vi "Digital_Bridge_3_kart.vi"() -> ()   [LabVIEW 2014] (continued)
                                frame 9 {
                                n4367 = Index Array(array=w3016, index (row)=w3015, index (col)=w3014) -> (element=w3013:dbl)
                                n4368 = Replace Array Subset(array=w3016, new element=w3013, index (row)=w3015, index (col)=w3014) -> (w3017:dbl[][])
                                }
                                }
                                n4369 = local write "Denge Kosulu y1_y2"(w2957) -> ()
                                }
                              }
                              frame 4, Default {
                                n4370 = for {
                                N: 10 -> [_]
                                tunnel: w3018 -> [w3020]
                                i -> [w3023]
                                n4371 = local read "Denge Kosulu y1_y2"() -> (w3022:dbl[][])
                                n4372 = case shown="0, Default" w3023 {
                                tunnel: w3023 -> [w3025 w3030 w3038 w3043 w3048 w3053 w3057 w3064 w3070 w3075]
                                tunnel: w3022 -> [w3026 w3032 w3037 w3042 w3047 w3052 w3055 w3062 w3071 w3076]
                                tunnel: [w3027 w3033 w3035 w3041 w3046 w3051 w3054 w3061 w3072 w3077] -> w3021
                                tunnel: w3020 -> [w3028 w3031 w3036 w3040 w3045 w3050 w3056 w3063 w3069 w3074]
                                frame 0, Default {
                                n4373 = Index Array(array=w3026, index (row)=w3025, index (col)=w3028) -> (element=w3024:dbl)
                                n4374 = Replace Array Subset(array=w3026, new element=w3024, index (row)=w3025, index (col)=w3028) -> (w3027:dbl[][])
                                }
                                frame 1 {
                                n4375 = Index Array(array=w3032, index (row)=w3030, index (col)=w3031) -> (element=w3029:dbl)
                                n4376 = Replace Array Subset(array=w3032, new element=w3029, index (row)=w3030, index (col)=w3031) -> (w3033:dbl[][])
                                }
                                frame 2 {
                                n4377 = Index Array(array=w3037, index (row)=w3038, index (col)=w3036) -> (element=w3034:dbl)
                                n4378 = Replace Array Subset(array=w3037, new element=w3034, index (row)=w3038, index (col)=w3036) -> (w3035:dbl[][])
                                }
                                frame 3 {
                                n4379 = Index Array(array=w3042, index (row)=w3043, index (col)=w3040) -> (element=w3039:dbl)
                                n4380 = Replace Array Subset(array=w3042, new element=w3039, index (row)=w3043, index (col)=w3040) -> (w3041:dbl[][])
                                }
                                frame 4 {
                                n4381 = Index Array(array=w3047, index (row)=w3048, index (col)=w3045) -> (element=w3044:dbl)
                                n4382 = Replace Array Subset(array=w3047, new element=w3044, index (row)=w3048, index (col)=w3045) -> (w3046:dbl[][])
                                }
                                frame 5 {
                                n4383 = Index Array(array=w3052, index (row)=w3053, index (col)=w3050) -> (element=w3049:dbl)
                                n4384 = Replace Array Subset(array=w3052, new element=w3049, index (row)=w3053, index (col)=w3050) -> (w3051:dbl[][])
                                }
                                frame 6 {
                                n4385 = Index Array(array=w3055, index (row)=w3057, index (col)=w3056) -> (element=w3060:dbl)
                                n4386 = Multiply(x=w3060, y=2.0) -> (x*y=w3058:dbl)
                                n4387 = Replace Array Subset(array=w3055, new element=w3058, index (row)=w3057, index (col)=w3056) -> (w3054:dbl[][])
                                }
                                frame 7 {
                                n4388 = Index Array(array=w3062, index (row)=w3064, index (col)=w3063) -> (element=w3067:dbl)
                                n4389 = Multiply(x=w3067, y=2.0) -> (x*y=w3065:dbl)
                                n4390 = Replace Array Subset(array=w3062, new element=w3065, index (row)=w3064, index (col)=w3063) -> (w3061:dbl[][])
                                }
                                frame 8 {
                                n4391 = Index Array(array=w3071, index (row)=w3070, index (col)=w3069) -> (element=w3068:dbl)
                                n4392 = Replace Array Subset(array=w3071, new element=w3068, index (row)=w3070, index (col)=w3069) -> (w3072:dbl[][])
                                }
                                frame 9 {
                                n4393 = Index Array(array=w3076, index (row)=w3075, index (col)=w3074) -> (element=w3073:dbl)
                                n4394 = Replace Array Subset(array=w3076, new element=w3073, index (row)=w3075, index (col)=w3074) -> (w3077:dbl[][])
                                }
                                }
                                n4395 = local write "Denge Kosulu y1_y2"(w3021) -> ()
                                }
                              }
                              frame 5 {
                                n4396 = for {
                                N: 10 -> [_]
                                tunnel: w3078 -> [w3080]
                                i -> [w3083]
                                n4397 = local read "Denge Kosulu y1_y2"() -> (w3082:dbl[][])
                                n4398 = case shown="0, Default" w3083 {
                                tunnel: w3083 -> [w3084 w3091 w3102 w3107 w3112 w3117 w3122 w3127 w3132 w3136]
                                tunnel: w3082 -> [w3085 w3093 w3101 w3106 w3111 w3116 w3120 w3125 w3133 w3137]
                                tunnel: [w3086 w3094 w3099 w3105 w3110 w3115 w3119 w3124 w3134 w3138] -> w3081
                                tunnel: w3080 -> [w3087 w3092 w3100 w3104 w3109 w3114 w3121 w3126 w3131 w3135]
                                frame 0, Default {
                                n4399 = Index Array(array=w3085, index (row)=w3084, index (col)=w3087) -> (element=w3090:dbl)
                                n4400 = Multiply(x=w3090, y=2.0) -> (x*y=w3088:dbl)
                                n4401 = Replace Array Subset(array=w3085, new element=w3088, index (row)=w3084, index (col)=w3087) -> (w3086:dbl[][])
                                }
                                frame 1 {
                                n4402 = Index Array(array=w3093, index (row)=w3091, index (col)=w3092) -> (element=w3097:dbl)
                                n4403 = Multiply(x=w3097, y=2.0) -> (x*y=w3095:dbl)
                                n4404 = Replace Array Subset(array=w3093, new element=w3095, index (row)=w3091, index (col)=w3092) -> (w3094:dbl[][])
                                }
                                frame 2 {
                                n4405 = Index Array(array=w3101, index (row)=w3102, index (col)=w3100) -> (element=w3098:dbl)
                                n4406 = Replace Array Subset(array=w3101, new element=w3098, index (row)=w3102, index (col)=w3100) -> (w3099:dbl[][])
                                }
                                frame 3 {
                                n4407 = Index Array(array=w3106, index (row)=w3107, index (col)=w3104) -> (element=w3103:dbl)
                                n4408 = Replace Array Subset(array=w3106, new element=w3103, index (row)=w3107, index (col)=w3104) -> (w3105:dbl[][])
                                }
                                frame 4 {
                                n4409 = Index Array(array=w3111, index (row)=w3112, index (col)=w3109) -> (element=w3108:dbl)
                                n4410 = Replace Array Subset(array=w3111, new element=w3108, index (row)=w3112, index (col)=w3109) -> (w3110:dbl[][])
                                }
                                frame 5 {
                                n4411 = Index Array(array=w3116, index (row)=w3117, index (col)=w3114) -> (element=w3113:dbl)
                                n4412 = Replace Array Subset(array=w3116, new element=w3113, index (row)=w3117, index (col)=w3114) -> (w3115:dbl[][])
                                }
                                frame 6 {
                                n4413 = Index Array(array=w3120, index (row)=w3122, index (col)=w3121) -> (element=w3118:dbl)
                                n4414 = Replace Array Subset(array=w3120, new element=w3118, index (row)=w3122, index (col)=w3121) -> (w3119:dbl[][])
                                }
                                frame 7 {
                                n4415 = Index Array(array=w3125, index (row)=w3127, index (col)=w3126) -> (element=w3123:dbl)
                                n4416 = Replace Array Subset(array=w3125, new element=w3123, index (row)=w3127, index (col)=w3126) -> (w3124:dbl[][])
                                }
                                frame 8 {
                                n4417 = Index Array(array=w3133, index (row)=w3132, index (col)=w3131) -> (element=w3130:dbl)
                                n4418 = Multiply(x=w3130, y=2.0) -> (x*y=w3128:dbl)
                                n4419 = Replace Array Subset(array=w3133, new element=w3128, index (row)=w3132, index (col)=w3131) -> (w3134:dbl[][])
                                }
                                frame 9 {
                                n4420 = Index Array(array=w3137, index (row)=w3136, index (col)=w3135) -> (element=w3141:dbl)
                                n4421 = Multiply(x=w3141, y=2.0) -> (x*y=w3139:dbl)
                                n4422 = Replace Array Subset(array=w3137, new element=w3139, index (row)=w3136, index (col)=w3135) -> (w3138:dbl[][])
                                }
                                }
                                n4423 = local write "Denge Kosulu y1_y2"(w3081) -> ()
                                }
                              }
                            }
                          }
                        }
                        n4424 = Equal?(x=w2179, y=0.0) -> (x = y?=w2177:bool)
                        n4425 = case shown="True" w2177 {
                          tunnel: [w2182 w2184] -> w2176
                          frame False {
                            n4426 = local read "frekans index"() -> (w2183:dbl)
                            n4427 = Decrement(x=w2183) -> (x-1=w2182:dbl)
                          }
                          frame True {
                            n4428 = local read "Frekanslar"() -> (w2186:dbl[])
                            n4429 = Array Size(array=w2186) -> (size(s)=w2187:i32)
                            n4430 = Decrement(x=w2187) -> (x-1=w2185:i32)
                            n4431 = To Double Precision Float(number=w2185) -> (double precision float=w2184:dbl)
                          }
                        }
                      }
                      frame True {
                        n4432 = flat-sequence {
                          tunnel: w3142 -> [w3155]
                          tunnel: [w3155] -> w3147
                          tunnel: w3147 -> [w3476]
                          tunnel: [w3476] -> w3146
                          tunnel: w3146 -> [w3797]
                          frame #0 {
                            n4433 = for {
                              N: 5 -> [_]
                              tunnel: w3155 -> [w3158]
                              i -> [w3157]
                              n4434 = Increment(x=w3157) -> (x+1=w3156:i32)
                              n4435 = case shown="1" w3156 {
                                tunnel: w3158 -> [w3159 w3223 w3287 w3351 w3411]
                                frame 1 {
                                n4436 = for {
                                N: 10 -> [_]
                                tunnel: w3159 -> [w3161]
                                i -> [w3164]
                                n4437 = local read "Denge Kosulu x2_y2"() -> (w3163:dbl[][])
                                n4438 = case shown="5" w3164 {
                                tunnel: w3164 -> [w3165 w3172 w3183 w3188 w3193 w3198 w3203 w3208 w3213 w3217]
                                tunnel: w3163 -> [w3166 w3174 w3182 w3187 w3192 w3197 w3201 w3206 w3214 w3218]
                                tunnel: [w3167 w3175 w3180 w3186 w3191 w3196 w3200 w3205 w3215 w3219] -> w3162
                                tunnel: w3161 -> [w3168 w3173 w3181 w3185 w3190 w3195 w3202 w3207 w3212 w3216]
                                frame 0, Default {
                                n4439 = Index Array(array=w3166, index (row)=w3165, index (col)=w3168) -> (element=w3171:dbl)
                                n4440 = Multiply(x=w3171, y=2.0) -> (x*y=w3169:dbl)
                                n4441 = Replace Array Subset(array=w3166, new element=w3169, index (row)=w3165, index (col)=w3168) -> (w3167:dbl[][])
                                }
                                frame 1 {
                                n4442 = Index Array(array=w3174, index (row)=w3172, index (col)=w3173) -> (element=w3178:dbl)
                                n4443 = Multiply(x=w3178, y=2.0) -> (x*y=w3176:dbl)
                                n4444 = Replace Array Subset(array=w3174, new element=w3176, index (row)=w3172, index (col)=w3173) -> (w3175:dbl[][])
                                }
                                frame 2 {
                                n4445 = Index Array(array=w3182, index (row)=w3183, index (col)=w3181) -> (element=w3179:dbl)
                                n4446 = Replace Array Subset(array=w3182, new element=w3179, index (row)=w3183, index (col)=w3181) -> (w3180:dbl[][])
                                }
                                frame 3 {
                                n4447 = Index Array(array=w3187, index (row)=w3188, index (col)=w3185) -> (element=w3184:dbl)
                                n4448 = Replace Array Subset(array=w3187, new element=w3184, index (row)=w3188, index (col)=w3185) -> (w3186:dbl[][])
                                }
                                frame 4 {
                                n4449 = Index Array(array=w3192, index (row)=w3193, index (col)=w3190) -> (element=w3189:dbl)
                                n4450 = Replace Array Subset(array=w3192, new element=w3189, index (row)=w3193, index (col)=w3190) -> (w3191:dbl[][])
                                }
                                frame 5 {
                                n4451 = Index Array(array=w3197, index (row)=w3198, index (col)=w3195) -> (element=w3194:dbl)
                                n4452 = Replace Array Subset(array=w3197, new element=w3194, index (row)=w3198, index (col)=w3195) -> (w3196:dbl[][])
                                }
                                frame 6 {
                                n4453 = Index Array(array=w3201, index (row)=w3203, index (col)=w3202) -> (element=w3199:dbl)
                                n4454 = Replace Array Subset(array=w3201, new element=w3199, index (row)=w3203, index (col)=w3202) -> (w3200:dbl[][])
                                }
                                frame 7 {
                                n4455 = Index Array(array=w3206, index (row)=w3208, index (col)=w3207) -> (element=w3204:dbl)
                                n4456 = Replace Array Subset(array=w3206, new element=w3204, index (row)=w3208, index (col)=w3207) -> (w3205:dbl[][])
                                }
                                frame 8 {
                                n4457 = Index Array(array=w3214, index (row)=w3213, index (col)=w3212) -> (element=w3211:dbl)
                                n4458 = Multiply(x=w3211, y=2.0) -> (x*y=w3209:dbl)
                                n4459 = Replace Array Subset(array=w3214, new element=w3209, index (row)=w3213, index (col)=w3212) -> (w3215:dbl[][])
                                }
                                frame 9 {
                                n4460 = Index Array(array=w3218, index (row)=w3217, index (col)=w3216) -> (element=w3222:dbl)
                                n4461 = Multiply(x=w3222, y=2.0) -> (x*y=w3220:dbl)
                                n4462 = Replace Array Subset(array=w3218, new element=w3220, index (row)=w3217, index (col)=w3216) -> (w3219:dbl[][])
                                }
                                }
                                n4463 = local write "Denge Kosulu x2_y2"(w3162) -> ()
                                }
                                }
                                frame 2 {
                                n4464 = for {
                                N: 10 -> [_]
                                tunnel: w3223 -> [w3225]
                                i -> [w3228]
                                n4465 = local read "Denge Kosulu x2_y2"() -> (w3227:dbl[][])
                                n4466 = case shown="7" w3228 {
                                tunnel: w3228 -> [w3230 w3235 w3242 w3249 w3256 w3263 w3271 w3276 w3279 w3284]
                                tunnel: w3227 -> [w3231 w3237 w3241 w3248 w3255 w3262 w3269 w3274 w3280 w3285]
                                tunnel: [w3232 w3238 w3239 w3247 w3254 w3261 w3268 w3273 w3281 w3286] -> w3226
                                tunnel: w3225 -> [w3233 w3236 w3240 w3246 w3253 w3260 w3270 w3275 w3278 w3283]
                                frame 0, Default {
                                n4467 = Index Array(array=w3231, index (row)=w3230, index (col)=w3233) -> (element=w3229:dbl)
                                n4468 = Replace Array Subset(array=w3231, new element=w3229, index (row)=w3230, index (col)=w3233) -> (w3232:dbl[][])
                                }
                                frame 1 {
                                n4469 = Index Array(array=w3237, index (row)=w3235, index (col)=w3236) -> (element=w3234:dbl)
                                n4470 = Replace Array Subset(array=w3237, new element=w3234, index (row)=w3235, index (col)=w3236) -> (w3238:dbl[][])
                                }
                                frame 2 {
                                n4471 = Index Array(array=w3241, index (row)=w3242, index (col)=w3240) -> (element=w3245:dbl)
                                n4472 = Multiply(x=w3245, y=2.0) -> (x*y=w3243:dbl)
                                n4473 = Replace Array Subset(array=w3241, new element=w3243, index (row)=w3242, index (col)=w3240) -> (w3239:dbl[][])
                                }
                                frame 3 {
                                n4474 = Index Array(array=w3248, index (row)=w3249, index (col)=w3246) -> (element=w3252:dbl)
                                n4475 = Multiply(x=w3252, y=2.0) -> (x*y=w3250:dbl)
                                n4476 = Replace Array Subset(array=w3248, new element=w3250, index (row)=w3249, index (col)=w3246) -> (w3247:dbl[][])
                                }
                                frame 4 {
                                n4477 = Index Array(array=w3255, index (row)=w3256, index (col)=w3253) -> (element=w3259:dbl)
                                n4478 = Multiply(x=w3259, y=2.0) -> (x*y=w3257:dbl)
                                n4479 = Replace Array Subset(array=w3255, new element=w3257, index (row)=w3256, index (col)=w3253) -> (w3254:dbl[][])
                                }
                                frame 5 {
                                n4480 = Index Array(array=w3262, index (row)=w3263, index (col)=w3260) -> (element=w3266:dbl)
                                n4481 = Multiply(x=w3266, y=2.0) -> (x*y=w3264:dbl)
                                n4482 = Replace Array Subset(array=w3262, new element=w3264, index (row)=w3263, index (col)=w3260) -> (w3261:dbl[][])
                                }
                                frame 6 {
                                n4483 = Index Array(array=w3269, index (row)=w3271, index (col)=w3270) -> (element=w3267:dbl)
                                n4484 = Replace Array Subset(array=w3269, new element=w3267, index (row)=w3271, index (col)=w3270) -> (w3268:dbl[][])
                                }
                                frame 7 {
                                n4485 = Index Array(array=w3274, index (row)=w3276, index (col)=w3275) -> (element=w3272:dbl)
                                n4486 = Replace Array Subset(array=w3274, new element=w3272, index (row)=w3276, index (col)=w3275) -> (w3273:dbl[][])
                                }
                                frame 8 {
                                n4487 = Index Array(array=w3280, index (row)=w3279, index (col)=w3278) -> (element=w3277:dbl)
                                n4488 = Replace Array Subset(array=w3280, new element=w3277, index (row)=w3279, index (col)=w3278) -> (w3281:dbl[][])
                                }
                                frame 9 {
                                n4489 = Index Array(array=w3285, index (row)=w3284, index (col)=w3283) -> (element=w3282:dbl)
                                n4490 = Replace Array Subset(array=w3285, new element=w3282, index (row)=w3284, index (col)=w3283) -> (w3286:dbl[][])
                                }
                                }
                                n4491 = local write "Denge Kosulu x2_y2"(w3226) -> ()
                                }
                                }
                                frame 3 {
                                n4492 = for {
                                N: 10 -> [_]
                                tunnel: w3287 -> [w3289]
                                i -> [w3292]
                                n4493 = local read "Denge Kosulu x2_y2"() -> (w3291:dbl[][])
                                n4494 = case shown="6" w3292 {
                                tunnel: w3292 -> [w3294 w3299 w3306 w3313 w3320 w3327 w3335 w3340 w3343 w3348]
                                tunnel: w3291 -> [w3295 w3301 w3305 w3312 w3319 w3326 w3333 w3338 w3344 w3349]
                                tunnel: [w3296 w3302 w3303 w3311 w3318 w3325 w3332 w3337 w3345 w3350] -> w3290
                                tunnel: w3289 -> [w3297 w3300 w3304 w3310 w3317 w3324 w3334 w3339 w3342 w3347]
                                frame 0, Default {
                                n4495 = Index Array(array=w3295, index (row)=w3294, index (col)=w3297) -> (element=w3293:dbl)
                                n4496 = Replace Array Subset(array=w3295, new element=w3293, index (row)=w3294, index (col)=w3297) -> (w3296:dbl[][])
                                }
                                frame 1 {
                                n4497 = Index Array(array=w3301, index (row)=w3299, index (col)=w3300) -> (element=w3298:dbl)
                                n4498 = Replace Array Subset(array=w3301, new element=w3298, index (row)=w3299, index (col)=w3300) -> (w3302:dbl[][])
                                }
                                frame 2 {
                                n4499 = Index Array(array=w3305, index (row)=w3306, index (col)=w3304) -> (element=w3309:dbl)
                                n4500 = Multiply(x=w3309, y=2.0) -> (x*y=w3307:dbl)
                                n4501 = Replace Array Subset(array=w3305, new element=w3307, index (row)=w3306, index (col)=w3304) -> (w3303:dbl[][])
                                }
                                frame 3 {
                                n4502 = Index Array(array=w3312, index (row)=w3313, index (col)=w3310) -> (element=w3316:dbl)
                                n4503 = Multiply(x=w3316, y=2.0) -> (x*y=w3314:dbl)
                                n4504 = Replace Array Subset(array=w3312, new element=w3314, index (row)=w3313, index (col)=w3310) -> (w3311:dbl[][])
                                }
                                frame 4 {
                                n4505 = Index Array(array=w3319, index (row)=w3320, index (col)=w3317) -> (element=w3323:dbl)
                                n4506 = Multiply(x=w3323, y=2.0) -> (x*y=w3321:dbl)
                                n4507 = Replace Array Subset(array=w3319, new element=w3321, index (row)=w3320, index (col)=w3317) -> (w3318:dbl[][])
                                }
                                frame 5 {
                                n4508 = Index Array(array=w3326, index (row)=w3327, index (col)=w3324) -> (element=w3330:dbl)
                                n4509 = Multiply(x=w3330, y=2.0) -> (x*y=w3328:dbl)
                                n4510 = Replace Array Subset(array=w3326, new element=w3328, index (row)=w3327, index (col)=w3324) -> (w3325:dbl[][])
                                }
                                frame 6 {
                                n4511 = Index Array(array=w3333, index (row)=w3335, index (col)=w3334) -> (element=w3331:dbl)
                                n4512 = Replace Array Subset(array=w3333, new element=w3331, index (row)=w3335, index (col)=w3334) -> (w3332:dbl[][])
                                }
                                frame 7 {
                                n4513 = Index Array(array=w3338, index (row)=w3340, index (col)=w3339) -> (element=w3336:dbl)
                                n4514 = Replace Array Subset(array=w3338, new element=w3336, index (row)=w3340, index (col)=w3339) -> (w3337:dbl[][])
                                }
                                frame 8 {
                                n4515 = Index Array(array=w3344, index (row)=w3343, index (col)=w3342) -> (element=w3341:dbl)
                                n4516 = Replace Array Subset(array=w3344, new element=w3341, index (row)=w3343, index (col)=w3342) -> (w3345:dbl[][])
                                }
                                frame 9 {
                                n4517 = Index Array(array=w3349, index (row)=w3348, index (col)=w3347) -> (element=w3346:dbl)
                                n4518 = Replace Array Subset(array=w3349, new element=w3346, index (row)=w3348, index (col)=w3347) -> (w3350:dbl[][])
                                }
                                }
                                n4519 = local write "Denge Kosulu x2_y2"(w3290) -> ()
                                }
                                }
                                frame 4, Default {
                                n4520 = for {
                                N: 10 -> [_]
                                tunnel: w3351 -> [w3353]
                                i -> [w3356]
                                n4521 = local read "Denge Kosulu x2_y2"() -> (w3355:dbl[][])
                                n4522 = case shown="6" w3356 {
                                tunnel: w3356 -> [w3358 w3363 w3371 w3376 w3381 w3386 w3390 w3397 w3403 w3408]
                                tunnel: w3355 -> [w3359 w3365 w3370 w3375 w3380 w3385 w3388 w3395 w3404 w3409]
                                tunnel: [w3360 w3366 w3368 w3374 w3379 w3384 w3387 w3394 w3405 w3410] -> w3354
                                tunnel: w3353 -> [w3361 w3364 w3369 w3373 w3378 w3383 w3389 w3396 w3402 w3407]
                                frame 0, Default {
                                n4523 = Index Array(array=w3359, index (row)=w3358, index (col)=w3361) -> (element=w3357:dbl)
                                n4524 = Replace Array Subset(array=w3359, new element=w3357, index (row)=w3358, index (col)=w3361) -> (w3360:dbl[][])
                                }
                                frame 1 {
                                n4525 = Index Array(array=w3365, index (row)=w3363, index (col)=w3364) -> (element=w3362:dbl)
                                n4526 = Replace Array Subset(array=w3365, new element=w3362, index (row)=w3363, index (col)=w3364) -> (w3366:dbl[][])
                                }
                                frame 2 {
                                n4527 = Index Array(array=w3370, index (row)=w3371, index (col)=w3369) -> (element=w3367:dbl)
                                n4528 = Replace Array Subset(array=w3370, new element=w3367, index (row)=w3371, index (col)=w3369) -> (w3368:dbl[][])
                                }
                                frame 3 {
                                n4529 = Index Array(array=w3375, index (row)=w3376, index (col)=w3373) -> (element=w3372:dbl)
                                n4530 = Replace Array Subset(array=w3375, new element=w3372, index (row)=w3376, index (col)=w3373) -> (w3374:dbl[][])
                                }
                                frame 4 {
                                n4531 = Index Array(array=w3380, index (row)=w3381, index (col)=w3378) -> (element=w3377:dbl)
                                n4532 = Replace Array Subset(array=w3380, new element=w3377, index (row)=w3381, index (col)=w3378) -> (w3379:dbl[][])
                                }
                                frame 5 {
                                n4533 = Index Array(array=w3385, index (row)=w3386, index (col)=w3383) -> (element=w3382:dbl)
                                n4534 = Replace Array Subset(array=w3385, new element=w3382, index (row)=w3386, index (col)=w3383) -> (w3384:dbl[][])
                                }
                                frame 6 {
                                n4535 = Index Array(array=w3388, index (row)=w3390, index (col)=w3389) -> (element=w3393:dbl)
                                n4536 = Multiply(x=w3393, y=2.0) -> (x*y=w3391:dbl)
                                n4537 = Replace Array Subset(array=w3388, new element=w3391, index (row)=w3390, index (col)=w3389) -> (w3387:dbl[][])
                                }
                                frame 7 {
                                n4538 = Index Array(array=w3395, index (row)=w3397, index (col)=w3396) -> (element=w3400:dbl)
                                n4539 = Multiply(x=w3400, y=2.0) -> (x*y=w3398:dbl)
                                n4540 = Replace Array Subset(array=w3395, new element=w3398, index (row)=w3397, index (col)=w3396) -> (w3394:dbl[][])
                                }
                                frame 8 {
                                n4541 = Index Array(array=w3404, index (row)=w3403, index (col)=w3402) -> (element=w3401:dbl)
                                n4542 = Replace Array Subset(array=w3404, new element=w3401, index (row)=w3403, index (col)=w3402) -> (w3405:dbl[][])
                                }
                                frame 9 {
                                n4543 = Index Array(array=w3409, index (row)=w3408, index (col)=w3407) -> (element=w3406:dbl)
                                n4544 = Replace Array Subset(array=w3409, new element=w3406, index (row)=w3408, index (col)=w3407) -> (w3410:dbl[][])
                                }
                                }
                                n4545 = local write "Denge Kosulu x2_y2"(w3354) -> ()
                                }
                                }
                                frame 5 {
                                n4546 = for {
                                N: 10 -> [_]
                                tunnel: w3411 -> [w3413]
                                i -> [w3416]
                                n4547 = local read "Denge Kosulu x2_y2"() -> (w3415:dbl[][])
                                n4548 = case shown="6" w3416 {
                                tunnel: w3416 -> [w3417 w3424 w3435 w3440 w3445 w3450 w3455 w3460 w3465 w3469]
                                tunnel: w3415 -> [w3418 w3426 w3434 w3439 w3444 w3449 w3453 w3458 w3466 w3470]
                                tunnel: [w3419 w3427 w3432 w3438 w3443 w3448 w3452 w3457 w3467 w3471] -> w3414
                                tunnel: w3413 -> [w3420 w3425 w3433 w3437 w3442 w3447 w3454 w3459 w3464 w3468]
                                frame 0, Default {
                                n4549 = Index Array(array=w3418, index (row)=w3417, index (col)=w3420) -> (element=w3423:dbl)
                                n4550 = Multiply(x=w3423, y=2.0) -> (x*y=w3421:dbl)
                                n4551 = Replace Array Subset(array=w3418, new element=w3421, index (row)=w3417, index (col)=w3420) -> (w3419:dbl[][])
                                }
                                frame 1 {
                                n4552 = Index Array(array=w3426, index (row)=w3424, index (col)=w3425) -> (element=w3430:dbl)
                                n4553 = Multiply(x=w3430, y=2.0) -> (x*y=w3428:dbl)
                                n4554 = Replace Array Subset(array=w3426, new element=w3428, index (row)=w3424, index (col)=w3425) -> (w3427:dbl[][])
                                }
                                frame 2 {
                                n4555 = Index Array(array=w3434, index (row)=w3435, index (col)=w3433) -> (element=w3431:dbl)
                                n4556 = Replace Array Subset(array=w3434, new element=w3431, index (row)=w3435, index (col)=w3433) -> (w3432:dbl[][])
                                }
                                frame 3 {
                                n4557 = Index Array(array=w3439, index (row)=w3440, index (col)=w3437) -> (element=w3436:dbl)
                                n4558 = Replace Array Subset(array=w3439, new element=w3436, index (row)=w3440, index (col)=w3437) -> (w3438:dbl[][])
                                }
                                frame 4 {
                                n4559 = Index Array(array=w3444, index (row)=w3445, index (col)=w3442) -> (element=w3441:dbl)
                                n4560 = Replace Array Subset(array=w3444, new element=w3441, index (row)=w3445, index (col)=w3442) -> (w3443:dbl[][])
                                }
                                frame 5 {
                                n4561 = Index Array(array=w3449, index (row)=w3450, index (col)=w3447) -> (element=w3446:dbl)
                                n4562 = Replace Array Subset(array=w3449, new element=w3446, index (row)=w3450, index (col)=w3447) -> (w3448:dbl[][])
                                }
                                frame 6 {
                                n4563 = Index Array(array=w3453, index (row)=w3455, index (col)=w3454) -> (element=w3451:dbl)
                                n4564 = Replace Array Subset(array=w3453, new element=w3451, index (row)=w3455, index (col)=w3454) -> (w3452:dbl[][])
                                }
                                frame 7 {
                                n4565 = Index Array(array=w3458, index (row)=w3460, index (col)=w3459) -> (element=w3456:dbl)
                                n4566 = Replace Array Subset(array=w3458, new element=w3456, index (row)=w3460, index (col)=w3459) -> (w3457:dbl[][])
                                }
                                frame 8 {
                                n4567 = Index Array(array=w3466, index (row)=w3465, index (col)=w3464) -> (element=w3463:dbl)
                                n4568 = Multiply(x=w3463, y=2.0) -> (x*y=w3461:dbl)
                                n4569 = Replace Array Subset(array=w3466, new element=w3461, index (row)=w3465, index (col)=w3464) -> (w3467:dbl[][])
                                }
                                frame 9 {
                                n4570 = Index Array(array=w3470, index (row)=w3469, index (col)=w3468) -> (element=w3474:dbl)
                                n4571 = Multiply(x=w3474, y=2.0) -> (x*y=w3472:dbl)
                                n4572 = Replace Array Subset(array=w3470, new element=w3472, index (row)=w3469, index (col)=w3468) -> (w3471:dbl[][])
                                }
                                }
                                n4573 = local write "Denge Kosulu x2_y2"(w3414) -> ()
                                }
                                }
                              }
                            }
                          }
                          frame #1 {
                            n4574 = for {
                              N: 5 -> [_]
                              tunnel: w3476 -> [w3479]
                              i -> [w3478]
                              n4575 = Increment(x=w3478) -> (x+1=w3477:i32)
                              n4576 = case shown="5" w3477 {
                                tunnel: w3479 -> [w3480 w3544 w3608 w3672 w3732]
                                frame 1 {
                                n4577 = for {
                                N: 10 -> [_]
                                tunnel: w3480 -> [w3482]
                                i -> [w3485]
                                n4578 = local read "Denge Kosulu x1_x2"() -> (w3484:dbl[][])
                                n4579 = case shown="0, Default" w3485 {
                                tunnel: w3485 -> [w3486 w3493 w3504 w3509 w3514 w3519 w3524 w3529 w3534 w3538]
                                tunnel: w3484 -> [w3487 w3495 w3503 w3508 w3513 w3518 w3522 w3527 w3535 w3539]
                                tunnel: [w3488 w3496 w3501 w3507 w3512 w3517 w3521 w3526 w3536 w3540] -> w3483
                                tunnel: w3482 -> [w3489 w3494 w3502 w3506 w3511 w3516 w3523 w3528 w3533 w3537]
                                frame 0, Default {
                                n4580 = Index Array(array=w3487, index (row)=w3486, index (col)=w3489) -> (element=w3492:dbl)
                                n4581 = Multiply(x=w3492, y=2.0) -> (x*y=w3490:dbl)
                                n4582 = Replace Array Subset(array=w3487, new element=w3490, index (row)=w3486, index (col)=w3489) -> (w3488:dbl[][])
                                }
                                frame 1 {
                                n4583 = Index Array(array=w3495, index (row)=w3493, index (col)=w3494) -> (element=w3499:dbl)
                                n4584 = Multiply(x=w3499, y=2.0) -> (x*y=w3497:dbl)
                                n4585 = Replace Array Subset(array=w3495, new element=w3497, index (row)=w3493, index (col)=w3494) -> (w3496:dbl[][])
                                }
                                frame 2 {
                                n4586 = Index Array(array=w3503, index (row)=w3504, index (col)=w3502) -> (element=w3500:dbl)
                                n4587 = Replace Array Subset(array=w3503, new element=w3500, index (row)=w3504, index (col)=w3502) -> (w3501:dbl[][])
                                }
                                frame 3 {
                                n4588 = Index Array(array=w3508, index (row)=w3509, index (col)=w3506) -> (element=w3505:dbl)
                                n4589 = Replace Array Subset(array=w3508, new element=w3505, index (row)=w3509, index (col)=w3506) -> (w3507:dbl[][])
                                }
                                frame 4 {
                                n4590 = Index Array(array=w3513, index (row)=w3514, index (col)=w3511) -> (element=w3510:dbl)
                                n4591 = Replace Array Subset(array=w3513, new element=w3510, index (row)=w3514, index (col)=w3511) -> (w3512:dbl[][])
                                }
                                frame 5 {
                                n4592 = Index Array(array=w3518, index (row)=w3519, index (col)=w3516) -> (element=w3515:dbl)
                                n4593 = Replace Array Subset(array=w3518, new element=w3515, index (row)=w3519, index (col)=w3516) -> (w3517:dbl[][])
                                }
                                frame 6 {
                                n4594 = Index Array(array=w3522, index (row)=w3524, index (col)=w3523) -> (element=w3520:dbl)
                                n4595 = Replace Array Subset(array=w3522, new element=w3520, index (row)=w3524, index (col)=w3523) -> (w3521:dbl[][])
                                }
                                frame 7 {
                                n4596 = Index Array(array=w3527, index (row)=w3529, index (col)=w3528) -> (element=w3525:dbl)
                                n4597 = Replace Array Subset(array=w3527, new element=w3525, index (row)=w3529, index (col)=w3528) -> (w3526:dbl[][])
                                }
                                frame 8 {
                                n4598 = Index Array(array=w3535, index (row)=w3534, index (col)=w3533) -> (element=w3532:dbl)
                                n4599 = Multiply(x=w3532, y=2.0) -> (x*y=w3530:dbl)
                                n4600 = Replace Array Subset(array=w3535, new element=w3530, index (row)=w3534, index (col)=w3533) -> (w3536:dbl[][])
                                }
                                frame 9 {
                                n4601 = Index Array(array=w3539, index (row)=w3538, index (col)=w3537) -> (element=w3543:dbl)
                                n4602 = Multiply(x=w3543, y=2.0) -> (x*y=w3541:dbl)
                                n4603 = Replace Array Subset(array=w3539, new element=w3541, index (row)=w3538, index (col)=w3537) -> (w3540:dbl[][])
                                }
                                }
                                n4604 = local write "Denge Kosulu x1_x2"(w3483) -> ()
                                }
                                }
                                frame 2 {
                                n4605 = for {
                                N: 10 -> [_]
                                tunnel: w3544 -> [w3546]
                                i -> [w3549]
                                n4606 = local read "Denge Kosulu x1_x2"() -> (w3548:dbl[][])
                                n4607 = case shown="0, Default" w3549 {
                                tunnel: w3549 -> [w3551 w3556 w3563 w3570 w3577 w3584 w3592 w3597 w3600 w3605]
                                tunnel: w3548 -> [w3552 w3558 w3562 w3569 w3576 w3583 w3590 w3595 w3601 w3606]
                                tunnel: [w3553 w3559 w3560 w3568 w3575 w3582 w3589 w3594 w3602 w3607] -> w3547
                                tunnel: w3546 -> [w3554 w3557 w3561 w3567 w3574 w3581 w3591 w3596 w3599 w3604]
                                frame 0, Default {
                                n4608 = Index Array(array=w3552, index (row)=w3551, index (col)=w3554) -> (element=w3550:dbl)
                                n4609 = Replace Array Subset(array=w3552, new element=w3550, index (row)=w3551, index (col)=w3554) -> (w3553:dbl[][])
                                }
                                frame 1 {
                                n4610 = Index Array(array=w3558, index (row)=w3556, index (col)=w3557) -> (element=w3555:dbl)
                                n4611 = Replace Array Subset(array=w3558, new element=w3555, index (row)=w3556, index (col)=w3557) -> (w3559:dbl[][])
                                }
                                frame 2 {
                                n4612 = Index Array(array=w3562, index (row)=w3563, index (col)=w3561) -> (element=w3566:dbl)
                                n4613 = Multiply(x=w3566, y=2.0) -> (x*y=w3564:dbl)
                                n4614 = Replace Array Subset(array=w3562, new element=w3564, index (row)=w3563, index (col)=w3561) -> (w3560:dbl[][])
                                }
                                frame 3 {
                                n4615 = Index Array(array=w3569, index (row)=w3570, index (col)=w3567) -> (element=w3573:dbl)
                                n4616 = Multiply(x=w3573, y=2.0) -> (x*y=w3571:dbl)
                                n4617 = Replace Array Subset(array=w3569, new element=w3571, index (row)=w3570, index (col)=w3567) -> (w3568:dbl[][])
                                }
                                frame 4 {
                                n4618 = Index Array(array=w3576, index (row)=w3577, index (col)=w3574) -> (element=w3580:dbl)
                                n4619 = Multiply(x=w3580, y=2.0) -> (x*y=w3578:dbl)
                                n4620 = Replace Array Subset(array=w3576, new element=w3578, index (row)=w3577, index (col)=w3574) -> (w3575:dbl[][])
                                }
                                frame 5 {
                                n4621 = Index Array(array=w3583, index (row)=w3584, index (col)=w3581) -> (element=w3587:dbl)
                                n4622 = Multiply(x=w3587, y=2.0) -> (x*y=w3585:dbl)
                                n4623 = Replace Array Subset(array=w3583, new element=w3585, index (row)=w3584, index (col)=w3581) -> (w3582:dbl[][])
                                }
                                frame 6 {
                                n4624 = Index Array(array=w3590, index (row)=w3592, index (col)=w3591) -> (element=w3588:dbl)
                                n4625 = Replace Array Subset(array=w3590, new element=w3588, index (row)=w3592, index (col)=w3591) -> (w3589:dbl[][])
                                }
                                frame 7 {
                                n4626 = Index Array(array=w3595, index (row)=w3597, index (col)=w3596) -> (element=w3593:dbl)
                                n4627 = Replace Array Subset(array=w3595, new element=w3593, index (row)=w3597, index (col)=w3596) -> (w3594:dbl[][])
                                }
                                frame 8 {
                                n4628 = Index Array(array=w3601, index (row)=w3600, index (col)=w3599) -> (element=w3598:dbl)
                                n4629 = Replace Array Subset(array=w3601, new element=w3598, index (row)=w3600, index (col)=w3599) -> (w3602:dbl[][])
                                }
                                frame 9 {
                                n4630 = Index Array(array=w3606, index (row)=w3605, index (col)=w3604) -> (element=w3603:dbl)
                                n4631 = Replace Array Subset(array=w3606, new element=w3603, index (row)=w3605, index (col)=w3604) -> (w3607:dbl[][])
                                }
                                }
                                n4632 = local write "Denge Kosulu x1_x2"(w3547) -> ()
                                }
                                }
                                frame 3 {
                                n4633 = for {
                                N: 10 -> [_]
                                tunnel: w3608 -> [w3610]
                                i -> [w3613]
                                n4634 = local read "Denge Kosulu x1_x2"() -> (w3612:dbl[][])
                                n4635 = case shown="0, Default" w3613 {
                                tunnel: w3613 -> [w3615 w3620 w3627 w3634 w3641 w3648 w3656 w3661 w3664 w3669]
                                tunnel: w3612 -> [w3616 w3622 w3626 w3633 w3640 w3647 w3654 w3659 w3665 w3670]
                                tunnel: [w3617 w3623 w3624 w3632 w3639 w3646 w3653 w3658 w3666 w3671] -> w3611
                                tunnel: w3610 -> [w3618 w3621 w3625 w3631 w3638 w3645 w3655 w3660 w3663 w3668]
                                frame 0, Default {
                                n4636 = Index Array(array=w3616, index (row)=w3615, index (col)=w3618) -> (element=w3614:dbl)
                                n4637 = Replace Array Subset(array=w3616, new element=w3614, index (row)=w3615, index (col)=w3618) -> (w3617:dbl[][])
                                }
                                frame 1 {
                                n4638 = Index Array(array=w3622, index (row)=w3620, index (col)=w3621) -> (element=w3619:dbl)
                                n4639 = Replace Array Subset(array=w3622, new element=w3619, index (row)=w3620, index (col)=w3621) -> (w3623:dbl[][])
                                }
                                frame 2 {
                                n4640 = Index Array(array=w3626, index (row)=w3627, index (col)=w3625) -> (element=w3630:dbl)
                                n4641 = Multiply(x=w3630, y=2.0) -> (x*y=w3628:dbl)
                                n4642 = Replace Array Subset(array=w3626, new element=w3628, index (row)=w3627, index (col)=w3625) -> (w3624:dbl[][])
                                }
                                frame 3 {
                                n4643 = Index Array(array=w3633, index (row)=w3634, index (col)=w3631) -> (element=w3637:dbl)
                                n4644 = Multiply(x=w3637, y=2.0) -> (x*y=w3635:dbl)
                                n4645 = Replace Array Subset(array=w3633, new element=w3635, index (row)=w3634, index (col)=w3631) -> (w3632:dbl[][])
                                }
                                frame 4 {
                                n4646 = Index Array(array=w3640, index (row)=w3641, index (col)=w3638) -> (element=w3644:dbl)
                                n4647 = Multiply(x=w3644, y=2.0) -> (x*y=w3642:dbl)
                                n4648 = Replace Array Subset(array=w3640, new element=w3642, index (row)=w3641, index (col)=w3638) -> (w3639:dbl[][])
                                }
                                frame 5 {
                                n4649 = Index Array(array=w3647, index (row)=w3648, index (col)=w3645) -> (element=w3651:dbl)
                                n4650 = Multiply(x=w3651, y=2.0) -> (x*y=w3649:dbl)
                                n4651 = Replace Array Subset(array=w3647, new element=w3649, index (row)=w3648, index (col)=w3645) -> (w3646:dbl[][])
                                }
                                frame 6 {
                                n4652 = Index Array(array=w3654, index (row)=w3656, index (col)=w3655) -> (element=w3652:dbl)
                                n4653 = Replace Array Subset(array=w3654, new element=w3652, index (row)=w3656, index (col)=w3655) -> (w3653:dbl[][])
                                }
                                frame 7 {
                                n4654 = Index Array(array=w3659, index (row)=w3661, index (col)=w3660) -> (element=w3657:dbl)
                                n4655 = Replace Array Subset(array=w3659, new element=w3657, index (row)=w3661, index (col)=w3660) -> (w3658:dbl[][])
                                }
                                frame 8 {
                                n4656 = Index Array(array=w3665, index (row)=w3664, index (col)=w3663) -> (element=w3662:dbl)
                                n4657 = Replace Array Subset(array=w3665, new element=w3662, index (row)=w3664, index (col)=w3663) -> (w3666:dbl[][])
                                }
                                frame 9 {
                                n4658 = Index Array(array=w3670, index (row)=w3669, index (col)=w3668) -> (element=w3667:dbl)
                                n4659 = Replace Array Subset(array=w3670, new element=w3667, index (row)=w3669, index (col)=w3668) -> (w3671:dbl[][])
                                }
                                }
                                n4660 = local write "Denge Kosulu x1_x2"(w3611) -> ()
                                }
                                }
                                frame 4, Default {
                                n4661 = for {
                                N: 10 -> [_]
                                tunnel: w3672 -> [w3674]
                                i -> [w3677]
                                n4662 = local read "Denge Kosulu x1_x2"() -> (w3676:dbl[][])
                                n4663 = case shown="0, Default" w3677 {
                                tunnel: w3677 -> [w3679 w3684 w3692 w3697 w3702 w3707 w3711 w3718 w3724 w3729]
                                tunnel: w3676 -> [w3680 w3686 w3691 w3696 w3701 w3706 w3709 w3716 w3725 w3730]
                                tunnel: [w3681 w3687 w3689 w3695 w3700 w3705 w3708 w3715 w3726 w3731] -> w3675
                                tunnel: w3674 -> [w3682 w3685 w3690 w3694 w3699 w3704 w3710 w3717 w3723 w3728]
                                frame 0, Default {
                                n4664 = Index Array(array=w3680, index (row)=w3679, index (col)=w3682) -> (element=w3678:dbl)
                                n4665 = Replace Array Subset(array=w3680, new element=w3678, index (row)=w3679, index (col)=w3682) -> (w3681:dbl[][])
                                }
                                frame 1 {
                                n4666 = Index Array(array=w3686, index (row)=w3684, index (col)=w3685) -> (element=w3683:dbl)
                                n4667 = Replace Array Subset(array=w3686, new element=w3683, index (row)=w3684, index (col)=w3685) -> (w3687:dbl[][])
                                }
                                frame 2 {
                                n4668 = Index Array(array=w3691, index (row)=w3692, index (col)=w3690) -> (element=w3688:dbl)
                                n4669 = Replace Array Subset(array=w3691, new element=w3688, index (row)=w3692, index (col)=w3690) -> (w3689:dbl[][])
                                }
                                frame 3 {
                                n4670 = Index Array(array=w3696, index (row)=w3697, index (col)=w3694) -> (element=w3693:dbl)
                                n4671 = Replace Array Subset(array=w3696, new element=w3693, index (row)=w3697, index (col)=w3694) -> (w3695:dbl[][])
                                }
                                frame 4 {
                                n4672 = Index Array(array=w3701, index (row)=w3702, index (col)=w3699) -> (element=w3698:dbl)
                                n4673 = Replace Array Subset(array=w3701, new element=w3698, index (row)=w3702, index (col)=w3699) -> (w3700:dbl[][])
                                }
                                frame 5 {
